vi "Insert Menu Separator.vi"(7 "menu tag":string, 9 "after item":string, 11 "Menu in":refnum<k9>) -> (1 "item tag":string, 3 "Menu out":refnum<k9>)   [LabVIEW 2020]
doc: "Insert a menu separator."
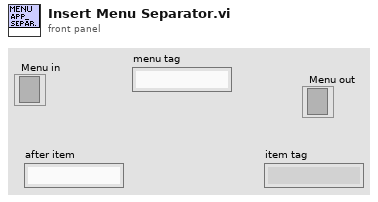
[diagram p1: front panel]
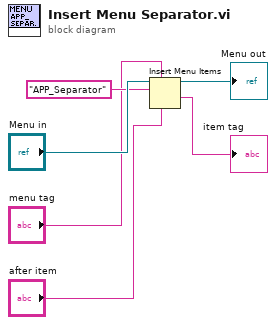
[diagram p0: block diagram]
diagram:
  n1 = Insert Menu Items(4:"after item", 5:"menu tag", 8:"APP_Separator", 9:"Menu in") -> (1:→"item tag":string, 3:→"Menu out":refnum<k9>)  [unwired: 2 in, 1 out]
